vi "Elevator_Hopper_code_untested.vi"() -> ()   [LabVIEW 2019]
uses:
  Control 2.ctl
  Control 3.ctl
  <vilib>/Rock Robotics/SystemInterfaces/DIO/FPGA_DIOPWMChannel.ctl
  <vilib>/Rock Robotics/WPI/PWM/WPI_PWMDeadband.ctl
  <vilib>/Rock Robotics/WPI/MotorControl/WPI_MotorControlType.ctl
  <vilib>/Rock Robotics/SystemInterfaces/DIO/FPGA_DIOChannel.ctl
  <vilib>/Rock Robotics/WPI/MotorControl/WPI_MotorControlDeviceRef.ctl
panel:
  in  "Elevator_Hopper":T1={"DeviceStatus"={"status"=FALSE, "code"=0, "source"=""}, "Type"=enum."PWM", "PWM"={"PWM Channel"=enum."Invalid", "DeadBand"={"Name"="", "maxPositivePwm"=0, "minPositivePwm"=0, "centerPwm"=0, "maxNegativePwm"=0, "minNegativePwm"=0, "angularRange"=0}}, "CAN"={"Device Number"=0, "SetOutput VI Ref"=variant(enum8{"Percent VBus", "Current", "Speed", "Position", "Voltage"} enum."Percent VBus"), "GetOutput VI Ref"=variant(refnum<k1> refnum), "Enable VI Ref"=variant(dbl 12.0), "Disable VI Ref"=variant(enum8{"Percent VBus", "Speed", "Position", "Slave", "Unchanged / Invalid"} enum."Percent VBus"), "Data"=variant}, "Invert"=FALSE, "DIO PWM"={"PWM \"Enable\" Channel"=enum."Invalid", "DIOChannel"=enum."Invalid", "PWM Rate"=0.0}}
  in  "Hopper Backwards":bool
  in  "Hopper Forwards":bool
  in  "Bakwards_Hopper":dbl
  in  "Stop_Hopper":dbl
  in  "Forwards_Hopper":dbl
  in  "Stop_elevator":dbl
  in  "Backwards_Elevator":dbl
  in  "Forwards_elevator":dbl
  in  "Elevator_Forwards_T/F":bool
  in  "Elevator_Backwards_T/F":bool
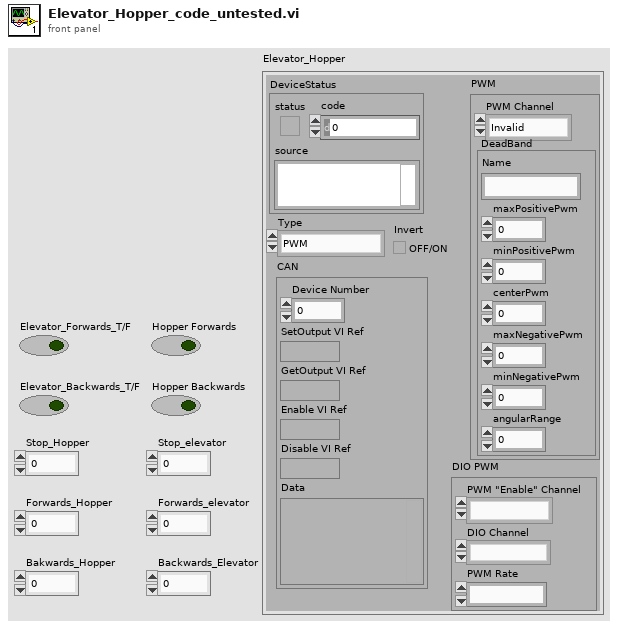
[diagram p1: front panel]
types:
  T1 = typedef "WPI_MotorControlDeviceRef.ctl" = cluster{"DeviceStatus":errorcluster, "Type":T2, "PWM":cluster{"PWM Channel":T3, "DeadBand":T4}, "CAN":cluster{"Device Number":u8, "SetOutput VI Ref":variant, "GetOutput VI Ref":variant, "Enable VI Ref":variant, "Disable VI Ref":variant, "Data":variant}, "Invert":bool, "DIO PWM":cluster{"PWM \"Enable\" Channel":T3, "DIOChannel":T5, "PWM Rate":dbl}}
  T2 = typedef "WPI_MotorControlType.ctl" = enum16{"PWM", "CAN", "DIO PWM"}
  T3 = typedef "FPGA_DIOPWMChannel.ctl" = enum8{"PWM 0", "PWM 1", "PWM 2", "PWM 3", "PWM 4", "PWM 5", "PWM 6", "PWM 7", "PWM 8", "PWM 9", "PWM MXP 0", "PWM MXP 1", "PWM MXP 2", "PWM MXP 3", "PWM MXP 4", "PWM MXP 5", "PWM MXP 6", "PWM MXP 7", "PWM MXP 8", "PWM MXP 9", "Invalid"}
  T4 = typedef "WPI_PWMDeadband.ctl" = cluster{"Name":string, "maxPositivePwm":i32, "minPositivePwm":i32, "centerPwm":i32, "maxNegativePwm":i32, "minNegativePwm":i32, "angularRange":u16}
  T5 = typedef "FPGA_DIOChannel.ctl" = enum8{"DIO 0", "DIO 1", "DIO 2", "DIO 3", "DIO 4", "DIO 5", "DIO 6", "DIO 7", "DIO 8", "DIO 9", "DIO MXP 0", "DIO MXP 1", "DIO MXP 2", "DIO MXP 3", "DIO MXP 4", "DIO MXP 5", "DIO MXP 6", "DIO MXP 7", "DIO MXP 8", "DIO MXP 9", "DIO MXP 10", "DIO MXP 11", "DIO MXP 12", "DIO MXP 13", "DIO MXP 14", "DIO MXP 15", "SPI Port CS1", "SPI Port CS2", "SPI Port CS3", "SPI Port MISO", "SPI Port MOSI", "Invalid"}
  T6 = typedef "Control 3.ctl" = enum16{"Elevator_forwards", "Elevator_Backwards", "Stop"}
  T7 = typedef "Control 2.ctl" = enum16{"Hopper_Forwards", "Hopper_Backwards", "Stop"}
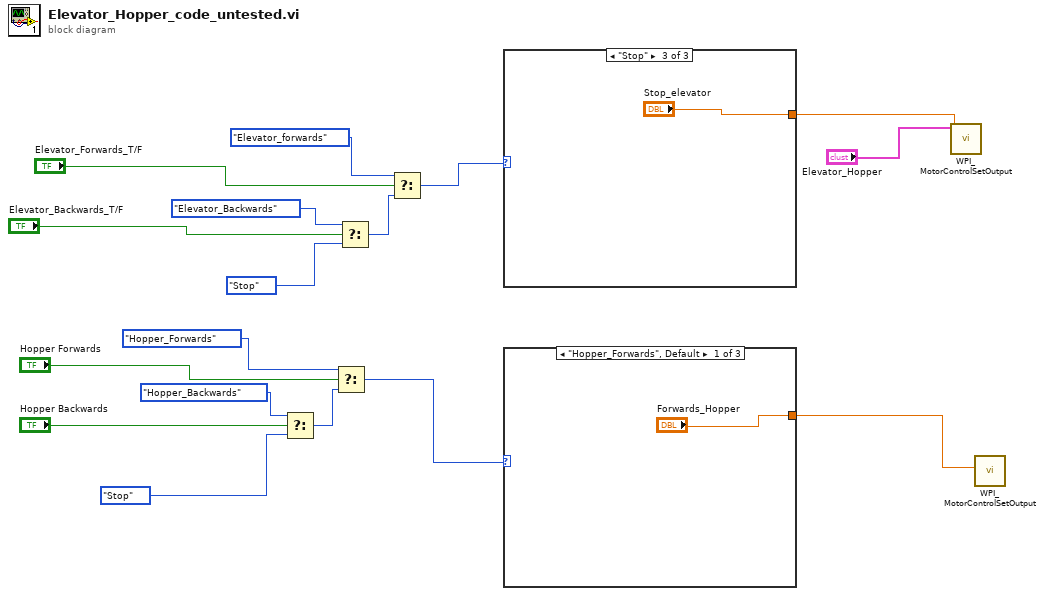
[diagram p0: block diagram]
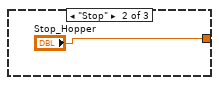
[diagram p2: hidden frame]
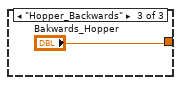
[diagram p3: hidden frame]
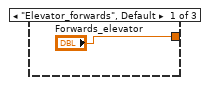
[diagram p4: hidden frame]
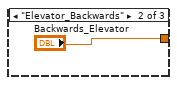
[diagram p5: hidden frame]
diagram:
  n1 = Select(t=Control_2."Hopper_Backwards", s="Hopper Backwards", f=Control_2."Stop") -> (s? t:f=w16:T7)
  n2 = Select(t=Control_2."Hopper_Forwards", s="Hopper Forwards", f=w16) -> (s? t:f=w8:T7)
  n3 = Select(t=Control_3."Elevator_Backwards", s="Elevator_Backwards_T/F", f=Control_3."Stop") -> (s? t:f=w17:T6)
  n4 = Select(t=Control_3."Elevator_forwards", s="Elevator_Forwards_T/F", f=w17) -> (s? t:f=w15:T6)
  n5 = case shown="\"Stop\"" w15 {
    tunnel: ["Forwards_elevator" "Backwards_Elevator" "Stop_elevator"] -> w4
    frame "Elevator_forwards", Default {
    }
    frame "Elevator_Backwards" {
    }
    frame "Stop" {
    }
  }
  n6 = case shown="\"Hopper_Forwards\", Default" w8 {
    tunnel: ["Forwards_Hopper" "Stop_Hopper" "Bakwards_Hopper"] -> w5
    frame "Hopper_Forwards", Default {
    }
    frame "Stop" {
    }
    frame "Hopper_Backwards" {
    }
  }
  n7 = call <vilib>:"WPI_MotorControlSetOutput.vi"("Output"=w4, "MotorControlDevRef"="Elevator_Hopper") -> ()  [unwired: 7 in, 3 out]
  n8 = call <vilib>:"WPI_MotorControlSetOutput.vi"("Output"=w5) -> ()  [unwired: 8 in, 3 out]
